vi "Draw Predicted Velocity.vi"(11 "State":T1) -> (3 "Predicted Velocity":cluster{dbl[], dbl[]}(graph))   [LabVIEW 2020]
uses:
  <vilib>/Analysis/Matrix/Datatypes/RealMatrix.ctl
  <vilib>/Analysis/baseanly.llb/Real A x B.vi
  <vilib>/Analysis/Matrix/NI_Matrix.lvlib
  <vilib>/Analysis/NI_AALBase.lvlib
  <vilib>/ptbypt/NI_PtbyPt.lvlib
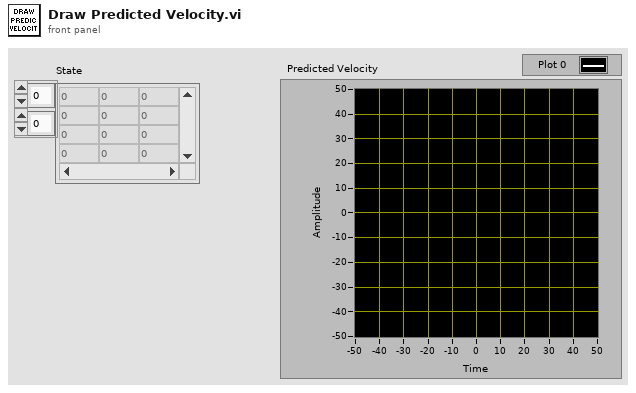
[diagram p1: front panel]
types:
  T1 = typedef "NI_Matrix.lvlib/RealMatrix.ctl" = dbl[][]
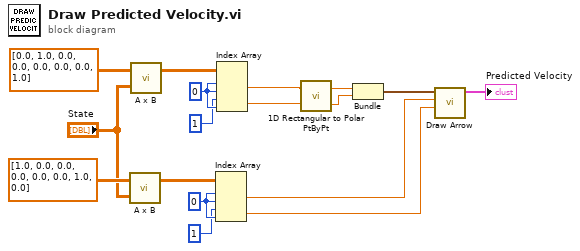
[diagram p0: block diagram]
diagram:
  w7 = 0 ("disabled index (col)")
  w16 = 0 ("disabled index (col)")
  n1 = call-poly <vilib>:"A x B.vi"("B"="State", "A"=T1 [[1.0, 0.0, 0.0, 0.0], [0.0, 0.0, 1.0, 0.0]] ("Initial Control Input")) -> ("A x B"=w8:T1)  [unwired: 1 out]
  n2 = call-poly <vilib>:"A x B.vi"("B"="State", "A"=T1 [[0.0, 1.0, 0.0, 0.0], [0.0, 0.0, 0.0, 1.0]] ("Initial Control Input")) -> ("A x B"=w17:T1)  [unwired: 1 out]
  n3 = Index Array(array=w8, index (row) #1=w7, index (col) #1=w7, index (row) #2=1 ("index (col)"), index (col) #2=w7) -> (element #1=w3:dbl, element #2=w2:dbl)
  n4 = Index Array(array=w17, index (row) #1=w16, index (col) #1=w16, index (row) #2=1 ("index (col)"), index (col) #2=w16) -> (element #1=w11:dbl, element #2=w13:dbl)
  n5 = call <vilib>:"1D Rectangular to Polar PtByPt.vi"("y"=w13, "x"=w11) -> ("phase"=w12:dbl, "magnitude"=w9:dbl)
  n6 = Bundle("magnitude"=w9, "phase"=w12) -> (w10:cluster{"magnitude":dbl, "phase":dbl})  [unwired: 1 in]
  n7 = call "Draw Arrow.vi"("Start Y"=w2, "Start X"=w3, "Vector"=w10) -> ("Points"=→"Predicted Velocity":cluster{dbl[], dbl[]})  [unwired: 6 in, 2 out]
